vi "SetupFile_Format.vi"(11 "DataCluster":T1={"Core"={"Current VI Reference"=refnum, "Close Panel on Exit?"=FALSE, "Exit"=FALSE, "Initialized?"=FALSE}, "Connections"={"cDAQ"={"Task"="ThermTask", "Connected"=FALSE, "Active"=FALSE, "ID"=""}, "Camera"={"Session"="", "Connected"=FALSE, "Active"=FALSE, "Placeholder"=refnum}, "PSU"={"Port"="", "Connected"=FALSE, "Active"=FALSE}, "Arduino"={"Port"="", "Connected"=FALSE, "Active"=FALSE}}, "Data Acquisition"={"Setup"={"Label"="Test Setup_1", "Operator"="", "Notes"="", "TempGrad"=1.0, "TargetTemp"=1.0, "Sample Volume"=1.0}, "Camera"={"Image"=refnum, "Save Image"=refnum, "Image Frequency"=20, "Rectangle"={"Left"=0, "Top"=0, "Right"=0, "Bottom"=0, "Rotation"=0.0}, "Calibration"={"Top Left"={"X"=0.0, "Y"=0.0}, "Top Right"={"X"=0.0, "Y"=0.0}, "Bottom Left"={"X"=0.0, "Y"=0.0}, "Bottom Right"={"X"=0.0, "Y"=0.0}, "Fixpoint"={"X"=0.0, "Y"=0.0}, "Scan Area"=0.0, "Fixpoint Area"=0.0, "Well Pixels"=[], "Valid"=FALSE}, "FocusPos"=0, "Display Mapping"=10, "Camera Mode"=10}, "Thermistor"={"Sample Size"=1, "Calibration"={"B0.100"=[3450.0, 3450.0, 3450.0, 3450.0, 3450.0, 3450.0, 3450.0, 3450.0], "R25"=[10.74, 10.74, 10.74, 10.74, 10.74, 10.74, 10.74, 10.74], "c"=[], "State"=[], "V_S"=10.0, "R_S"=10.0}, "Timing Mode"=14713}, "Partition"={"Data"=[["A", "35%", "", "", ""], ["B", "15%", "", "", ""], ["C", "5%", "", "", ""], ["D", "35%", "", "", ""], ["E", "Test sample", "", "", ""], ["F", "High Concentration", "", "", ""], ["G", "Low Concentration", "", "", ""], ["X", "Empty", "", "", ""]], "Cell Label"="F", "Cell Color"=5095150, "Height"=8, "Width"=12, "Grid"=[["A", "A", "A", "B", "B", "B", "B", "B", "B", "B", "B", "B"], ["A", "A", "A", "B", "B", "B", "B", "B", "B", "B", "B", "B"], ["A", "A", "A", "B", "B", "B", "B", "B", "B", "B", "B", "B"], ["A", "A", "A", "C", "C", "C", "D", "D", "D", "D", "D", "D"], ["A", "A", "A", "C", "C", "C", "D", "D", "D", "D", "D", "D"], ["A", "A", "A", "C", "C", "C", "E", "E", "F", "F", "G", "G"], ["A", "A", "A", "C", "C", "C", "E", "E", "F", "F", "G", "G"], ["A", "A", "A", "C", "C", "C", "E", "E", "F", "F", "G", "G"]]}, "Queue"={"Size"=1, "Queue"=refnum}, "Sample Rate"=60, "Active"=TRUE, "Ready"=TRUE, "Graph Mode"=0, "Gradient Buffer"=2}, "Control"={"Sample Rate"=1, "PID gains"={"proportional gain (Kc)"=1.0, "integral time (Ti, min)"=0.01, "derivative time (Td, min)"=0.0}}, "Manual Temp Control"={"TargetTemp"=1.0, "Mode"=0, "Active"=FALSE}} {"Manual Temp Control"."Mode" items=["Cool", "Heat"]; "Manual Temp Control"."TargetTemp" min=-40.0 max=40.0 step=0.5 format="%#_g °C"; "Control"."PID gains"."derivative time (Td, min)" format="%.3f"; "Control"."PID gains"."integral time (Ti, min)" format="%.3f"; "Control"."PID gains"."proportional gain (Kc)" format="%.3f"; "Control"."Sample Rate" min=1 max=20 step=1 format="%.0f Samples/sec"; "Data Acquisition"."Gradient Buffer" min=2 max=30 step=1; "Data Acquisition"."Graph Mode" items=["Thermistor Temperature", "Camera Temperature"]; "Data Acquisition"."Thermistor"."Timing Mode" items=["Automatic"=16097, "High Resolution"=10195, "High Speed"=14712, "Best 50 Hz Rejection"=14713, "Best 60 Hz Rejection"=14714, "Custom"=10137]; "Data Acquisition"."Thermistor"."Calibration"."R_S" min=0.1 max=1000.0 format="%#_g kOhm"; "Data Acquisition"."Thermistor"."Calibration"."V_S" min=5.0 max=48.0 format="%#_g V"; "Data Acquisition"."Thermistor"."Calibration"."R25" min=0.1 max=1000.0 format="%#_g kOhm"; "Data Acquisition"."Thermistor"."Calibration"."B0.100" min=100.0 max=10000.0 format="%#_g K"; "Data Acquisition"."Thermistor"."Sample Size" min=1 max=200; "Data Acquisition"."Sample Rate" min=20 max=240 format="%.0f samples/min"; "Data Acquisition"."Queue"."Size" min=1 max=200; "Data Acquisition"."Camera"."Camera Mode" items=["Temperature Linear", "Signal Linear"]; "Data Acquisition"."Camera"."Display Mapping" items=["Default"=10, "Most Significant Bits"=11, "Full Dynamic"=12, "Downshift"=13, "Given Range"=14, "90% Dynamic"=15, "Given Percent Range"=16]; "Data Acquisition"."Camera"."Calibration"."Fixpoint"."Y" format="%.2f"; "Data Acquisition"."Camera"."Calibration"."Fixpoint"."X" format="%.2f"; "Data Acquisition"."Camera"."Calibration"."Top Left"."Y" format="%.2f"; "Data Acquisition"."Camera"."Calibration"."Top Left"."X" format="%.2f"; "Data Acquisition"."Camera"."Calibration"."Top Right"."Y" format="%.2f"; "Data Acquisition"."Camera"."Calibration"."Top Right"."X" format="%.2f"; "Data Acquisition"."Camera"."Calibration"."Bottom Left"."Y" format="%.2f"; "Data Acquisition"."Camera"."Calibration"."Bottom Left"."X" format="%.2f"; "Data Acquisition"."Camera"."Calibration"."Bottom Right"."Y" format="%.2f"; "Data Acquisition"."Camera"."Calibration"."Bottom Right"."X" format="%.2f"; "Data Acquisition"."Camera"."Rectangle"."Rotation" min=-90.0 max=90.0 step=1.0 format="%.2f"; "Data Acquisition"."Camera"."Rectangle"."Left" scale=0.0..1024.0; "Data Acquisition"."Camera"."Rectangle"."Right" scale=0.0..1024.0; "Data Acquisition"."Camera"."Image Frequency" min=1 max=60 step=1; "Data Acquisition"."Setup"."Sample Volume" min=0.0 max=500.0 format="%#_g µL"; "Data Acquisition"."Setup"."TargetTemp" min=-40.0 max=40.0 step=0.5 format="%#_g °C"; "Data Acquisition"."Setup"."TempGrad" min=-100.0 max=100.0 step=0.1 format="%#_g °C/min"}) -> (2 "Partition":string[][](array[string])=[["Ice Nucleation Version", "0.0.0.1", "", "Partition", "Description", "", " ", "1", "2", "3", "4", "5", "6", "7", "8", "9", "10", "11", "12"], ["", "", "", "A", "35%", "", "A", "A", "A", "A", "B", "B", "B", "B", "B", "B", "B", "B", "B"], ["Sample:", "", "", "B", "15%", "", "B", "A", "A", "A", "B", "B", "B", "B", "B", "B", "B", "B", "B"], ["Label", "Test Setup_1", "", "C", "5%", "", "C", "A", "A", "A", "B", "B", "B", "B", "B", "B", "B", "B", "B"], ["Operator", "", "", "D", "35%", "", "D", "A", "A", "A", "C", "C", "C", "D", "D", "D", "D", "D", "D"], ["Date", "2021_07_12-12-50-49-038", "", "E", "Test sample", "", "E", "A", "A", "A", "C", "C", "C", "D", "D", "D", "D", "D", "D"], ["PCR type", "12x8", "", "F", "High Concentration", "", "F", "A", "A", "A", "C", "C", "C", "E", "E", "F", "F", "G", "G"], ["", "", "", "G", "Low Concentration", "", "G", "A", "A", "A", "C", "C", "C", "E", "E", "F", "F", "G", "G"], ["Sample volume [µL]", "1,00", "", "X", "Empty", "", "H", "A", "A", "A", "C", "C", "C", "E", "E", "F", "F", "G", "G"], ["Temperature Gradient [°C/min]", "1,00", "", "", "", "", "", "", "", "", "", "", "", "", "", "", "", "", ""], ["Target Temperature [°C] ", "1,00", "", "", "", "", "", "", "", "", "", "", "", "", "", "", "", "", ""], ["Starting Temp [°C]", "0,000000", "", "", "", "", "", "", "", "", "", "", "", "", "", "", "", "", ""], ["Ending Temp [°C]", "Ending_Temp", "", "", "", "", "", "", "", "", "", "", "", "", "", "", "", "", ""], ["Test Duration [mm:ss]", "Test_Duration", "", "", "", "", "", "", "", "", "", "", "", "", "", "", "", "", ""], ["", "", "", "", "", "", "", "", "", "", "", "", "", "", "", "", "", "", ""], ["PID setup:", "", "", "", "", "", "", "", "", "", "", "", "", "", "", "", "", "", ""], ["Proportional Gain", "1,000000", "", "", "", "", "", "", "", "", "", "", "", "", "", "", "", "", ""], ["Integral time (min)", "0,010000", "", "", "", "", "", "", "", "", "", "", "", "", "", "", "", "", ""], ["Derivative time (min)", "0,000000", "", "", "", "", "", "", "", "", "", "", "", "", "", "", "", "", ""], ["", "", "", "", "", "", "", "", "", "", "", "", "", "", "", "", "", "", ""], ["Calibration Values:", "\r", "", "", "", "", "", "", "", "", "", "", "", "", "", "", "", "", ""], ["B0_100", "", "", "", "", "", "", "", "", "", "", "", "", "", "", "", "", "", ""], ["R25", "", "", "", "", "", "", "", "", "", "", "", "", "", "", "", "", "", ""], ["", "", "", "", "", "", "", "", "", "", "", "", "", "", "", "", "", "", ""], ["Notes:", "", "", "", "", "", "", "", "", "", "", "", "", "", "", "", "", "", ""]], 3 "Array":string[][](array[string])=[["Ice Nucleation Version", "0.0.0.1", "", "Partition", "Description", "", " ", "1", "2", "3", "4", "5", "6", "7", "8", "9", "10", "11", "12"], ["", "", "", "A", "35%", "", "A", "A", "A", "A", "B", "B", "B", "B", "B", "B", "B", "B", "B"], ["Sample:", "", "", "B", "15%", "", "B", "A", "A", "A", "B", "B", "B", "B", "B", "B", "B", "B", "B"], ["Label", "Test Setup_1", "", "C", "5%", "", "C", "A", "A", "A", "B", "B", "B", "B", "B", "B", "B", "B", "B"], ["Operator", "", "", "D", "35%", "", "D", "A", "A", "A", "C", "C", "C", "D", "D", "D", "D", "D", "D"], ["Date", "2021_07_12-12-50-49-038", "", "E", "Test sample", "", "E", "A", "A", "A", "C", "C", "C", "D", "D", "D", "D", "D", "D"], ["PCR type", "12x8", "", "F", "High Concentration", "", "F", "A", "A", "A", "C", "C", "C", "E", "E", "F", "F", "G", "G"], ["", "", "", "G", "Low Concentration", "", "G", "A", "A", "A", "C", "C", "C", "E", "E", "F", "F", "G", "G"], ["Sample volume [µL]", "1,00", "", "X", "Empty", "", "H", "A", "A", "A", "C", "C", "C", "E", "E", "F", "F", "G", "G"], ["Temperature Gradient [°C/min]", "1,00", "", "", "", "", "", "", "", "", "", "", "", "", "", "", "", "", ""], ["Target Temperature [°C] ", "1,00", "", "", "", "", "", "", "", "", "", "", "", "", "", "", "", "", ""], ["Starting Temp [°C]", "0,000000", "", "", "", "", "", "", "", "", "", "", "", "", "", "", "", "", ""], ["Ending Temp [°C]", "Ending_Temp", "", "", "", "", "", "", "", "", "", "", "", "", "", "", "", "", ""], ["Test Duration [mm:ss]", "Test_Duration", "", "", "", "", "", "", "", "", "", "", "", "", "", "", "", "", ""], ["", "", "", "", "", "", "", "", "", "", "", "", "", "", "", "", "", "", ""], ["PID setup:", "", "", "", "", "", "", "", "", "", "", "", "", "", "", "", "", "", ""], ["Proportional Gain", "1,000000", "", "", "", "", "", "", "", "", "", "", "", "", "", "", "", "", ""], ["Integral time (min)", "0,010000", "", "", "", "", "", "", "", "", "", "", "", "", "", "", "", "", ""], ["Derivative time (min)", "0,000000", "", "", "", "", "", "", "", "", "", "", "", "", "", "", "", "", ""], ["", "", "", "", "", "", "", "", "", "", "", "", "", "", "", "", "", "", ""], ["Calibration Values:", "\r", "", "", "", "", "", "", "", "", "", "", "", "", "", "", "", "", ""], ["B0_100", "", "", "", "", "", "", "", "", "", "", "", "", "", "", "", "", "", ""], ["R25", "", "", "", "", "", "", "", "", "", "", "", "", "", "", "", "", "", ""], ["", "", "", "", "", "", "", "", "", "", "", "", "", "", "", "", "", "", ""], ["Notes:", "", "", "", "", "", "", "", "", "", "", "", "", "", "", "", "", "", ""]])   [LabVIEW 2024]
uses:
  DataCluster.ctl
  <vilib>/userDefined/High Color/IMAQdx.ctl
  <vilib>/vision/Image Controls.llb/IMAQ Image.ctl
panel:
  in  "Labels":string[](array[string])=["Ice Nucleation Version", "", "Sample:", "Label", "Operator", "Date", "PCR type", "", "Sample volume [µL]", "Temperature Gradient [°C/min]", "Target Temperature [°C] ", "Starting Temp [°C]", "Ending Temp [°C]", "Test Duration [mm:ss]", "", "PID setup:", "Proportional Gain", "Integral time (min)", "Derivative time (min)", "", "Calibration Values:", "B0_100", "R25", "R_S", "", "Notes:"]
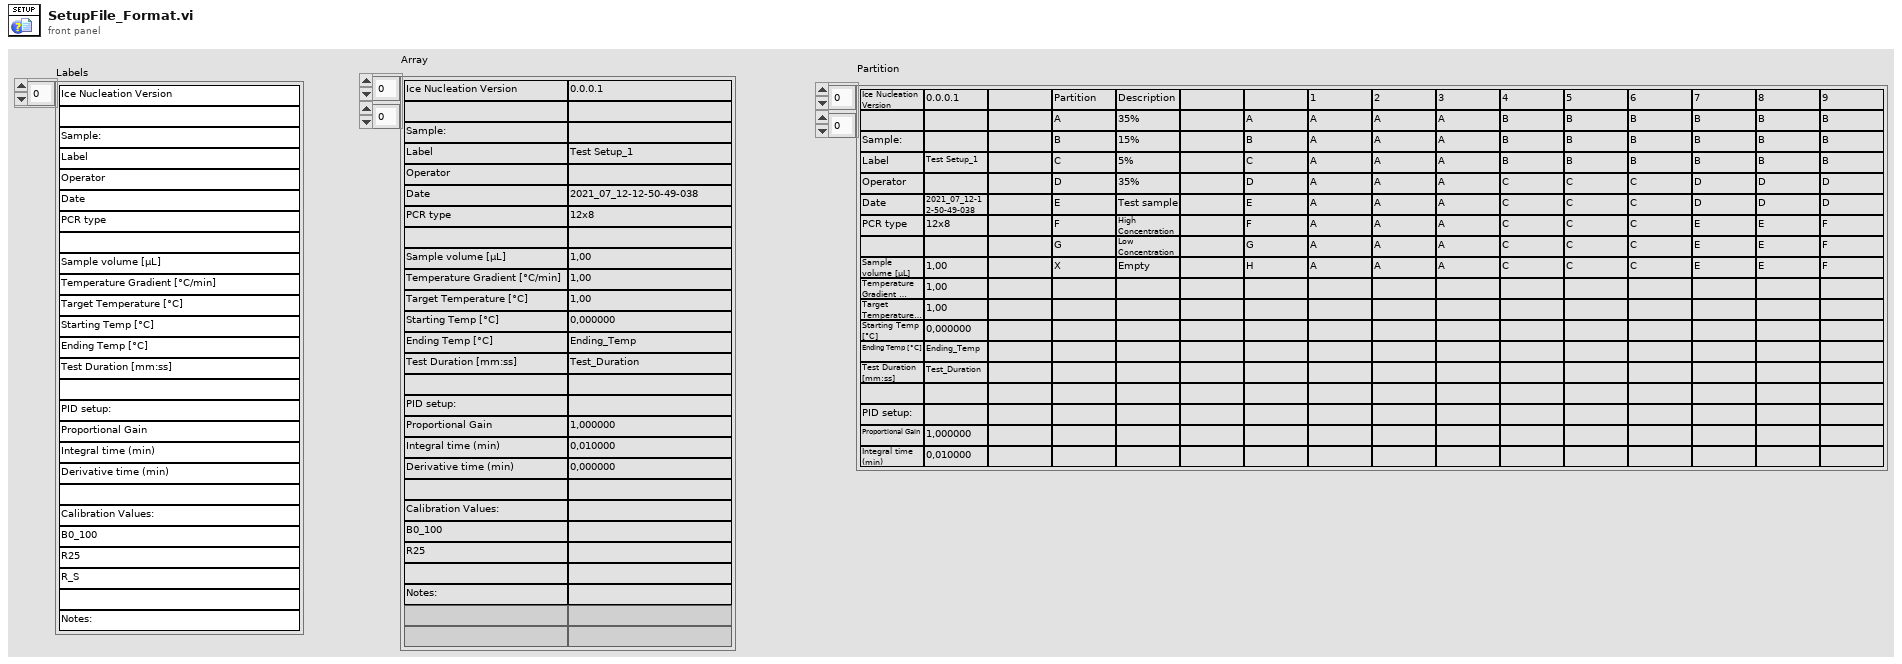
[diagram p1: front panel]
types:
  T1 = typedef "DataCluster.ctl" = cluster{"Core":cluster{"Current VI Reference":refnum<vi>, "Close Panel on Exit?":bool, "Exit":bool, "Initialized?":bool}, "Connections":cluster{"cDAQ":cluster{"Task":refnum<k21>, "Connected":bool, "Active":bool, "ID":string}, "Camera":cluster{"Session":T2, "Connected":bool, "Active":bool, "Placeholder":T3}, "PSU":cluster{"Port":refnum<visa-resource-name>, "Connected":bool, "Active":bool}, "Arduino":cluster{"Port":refnum<visa-resource-name>, "Connected":bool, "Active":bool}}, "Data Acquisition":cluster{"Setup":cluster{"Label":string, "Operator":string, "Notes":string, "TempGrad":dbl, "TargetTemp":dbl, "Sample Volume":dbl}, "Camera":cluster{"Image":T3, "Save Image":T3, "Image Frequency":i32, "Rectangle":T4, "Calibration":cluster{"Top Left":T5, "Top Right":T5, "Bottom Left":T5, "Bottom Right":T5, "Fixpoint":T5, "Scan Area":dbl, "Fixpoint Area":dbl, "Well Pixels":cluster{"X":i32, "Y":i32}[][], "Valid":bool}, "FocusPos":u32, "Display Mapping":u32, "Camera Mode":u32}, "Thermistor":cluster{"Sample Size":i32, "Calibration":cluster{"B0.100":dbl[], "R25":dbl[], "c":dbl[][], "State":bool[], "V_S":dbl, "R_S":dbl}, "Timing Mode":i32}, "Partition":cluster{"Data":string[][], "Cell Label":string, "Cell Color":u32, "Height":i32, "Width":i32, "Grid":string[][]}, "Queue":cluster{"Size":i32, "Queue":refnum<queue>}, "Sample Rate":i32, "Active":bool, "Ready":bool, "Graph Mode":u16, "Gradient Buffer":i32}, "Control":cluster{"Sample Rate":i32, "PID gains":cluster{"proportional gain (Kc)":dbl, "integral time (Ti, min)":dbl, "derivative time (Td, min)":dbl}}, "Manual Temp Control":cluster{"TargetTemp":dbl, "Mode":u16, "Active":bool}}
  T2 = typedef "IMAQdx.ctl" = refnum<k21>
  T3 = typedef "IMAQ Image.ctl" = refnum<image>
  T4 = typedef "IMAQ Rectangle" = cluster{"Left":i32, "Top":i32, "Right":i32, "Bottom":i32, "Rotation":dbl}
  T5 = typedef "IMAQ Point" = cluster{"X":sgl, "Y":sgl}
  T6 = cluster{"Label":string, "Operator":string, "Notes":string, "TempGrad":dbl, "TargetTemp":dbl, "Sample Volume":dbl}
  T7 = cluster{"proportional gain (Kc)":dbl, "integral time (Ti, min)":dbl, "derivative time (Td, min)":dbl}
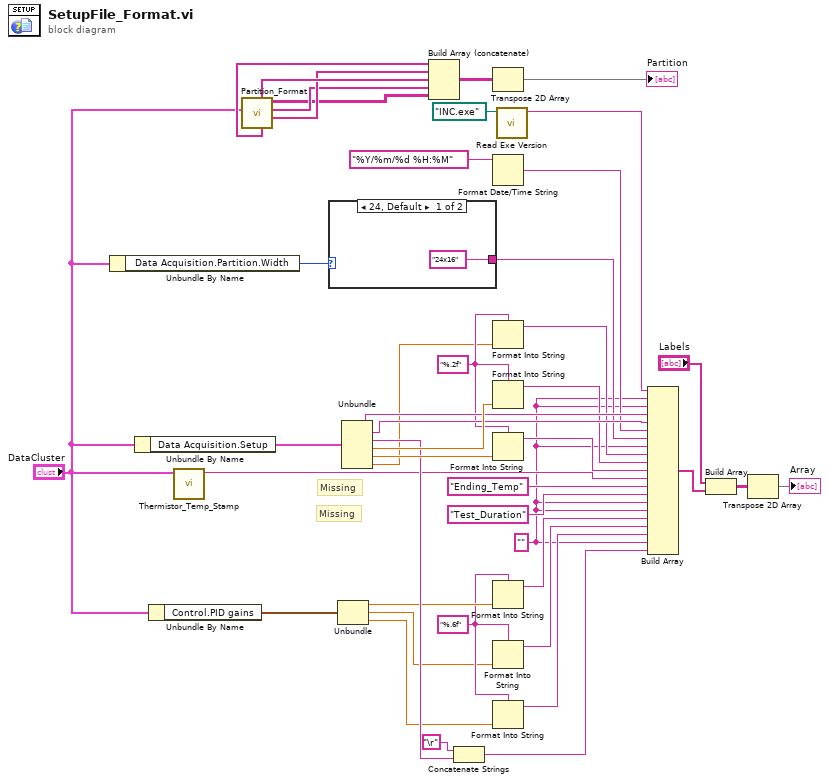
[diagram p0: block diagram]
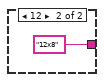
[diagram p2: hidden frame]
diagram:
  w27 = "%.6f" ("format string")
  w19 = "%.2f" ("format string")
  w9 = "" ("element")
  # "Missing"
  # "Missing"
  n1 = Unbundle By Name("DataCluster") -> ("Data Acquisition.Partition.Width"=w21:i32)
  n2 = Unbundle By Name("DataCluster") -> ("Data Acquisition.Setup"=w38:T6)
  n3 = Unbundle By Name("DataCluster") -> ("Control.PID gains"=w29:T7)
  n4 = call "Thermistor_Temp_Stamp.vi"("DataCluster"="DataCluster") -> ("mean temp"=w11:string)  [unwired: 9 in, 1 out]
  n5 = call "Partition_Format.vi"("input cluster"="DataCluster") -> ("Array 3"=w14:string[], "Alphabetical"=w13:string[], "Grid out"=w12:string[][], "Labels out"=w15:string[], "empty Element"=w16:string[])  [unwired: 6 in]
  n6 = case shown="24, Default" w21 {
    tunnel: ["24x16" ("element") "12x8" ("element")] -> w20
    frame 24, Default {
    }
    frame 12 {
    }
  }
  n7 = Unbundle(w29) -> ("proportional gain (Kc)"=w28:dbl, "integral time (Ti, min)"=w26:dbl, "derivative time (Td, min)"=w25:dbl)
  n8 = Unbundle(w38) -> ("Label"=w40:string, "Operator"=w35:string, "Notes"=w36:string, "TempGrad"=w41:dbl, "TargetTemp"=w42:dbl, "Sample Volume"=w17:dbl)
  n9 = Build Array (concatenate)(w15, w14, w16, w13, w12) -> (w43:string[][])
  n10 = Concatenate Strings("\r", w36) -> (w8:string)
  n11 = Transpose 2D Array(2D array=w43) -> (transposed array=→"Partition":string[][])
  n12 = Format Date/Time String(time format string (%c)="%Y/%m/%d %H:%M") -> (date/time string=w34:string)  [unwired: 2 in]
  n13 = Format Into String(format string=w19, w17) -> (resulting string=w18:string)  [unwired: 2 in, 1 out]
  n14 = Format Into String(format string=w19, w41) -> (resulting string=w32:string)  [unwired: 2 in, 1 out]
  n15 = Format Into String(format string=w19, w42) -> (resulting string=w31:string)  [unwired: 2 in, 1 out]
  n16 = Format Into String(format string=w27, w28) -> (resulting string=w24:string)  [unwired: 2 in, 1 out]
  n17 = Format Into String(format string=w27, w26) -> (resulting string=w23:string)  [unwired: 2 in, 1 out]
  n18 = Format Into String(format string=w27, w25) -> (resulting string=w22:string)  [unwired: 2 in, 1 out]
  n19 = call "Read Exe Version.vi"("Application name"=path "INC.exe") -> ("FileVersion"=w39:string)  [unwired: 7 in, 3 out]
  n20 = Build Array(w39, w9, w9, w40, w35, w34, w20, w9, w18, w32, w31, w11, "Ending_Temp" ("element"), "Test_Duration" ("element"), w9, w9, w24, w23, w22, w9, w8) -> (w5:string[])
  n21 = Build Array("Labels", w5) -> (w3:string[][])
  n22 = Transpose 2D Array(2D array=w3) -> (transposed array=→"Array":string[][])
